vi "Read controlTerminalRef.vi"(8 "error in (no error)":errorcluster, 11 "Terminal In":refnum<class "ControlTerminal.lvclass">) -> (0 "error out":errorcluster, 2 "terminalRef":refnum<vi>, 3 "Terminal Out":refnum<class "ControlTerminal.lvclass">)   [LabVIEW 2023, in "TLC_Scripto.lvlib" / "ControlTerminal.lvclass"]
uses:
  ControlTerminal.lvclass
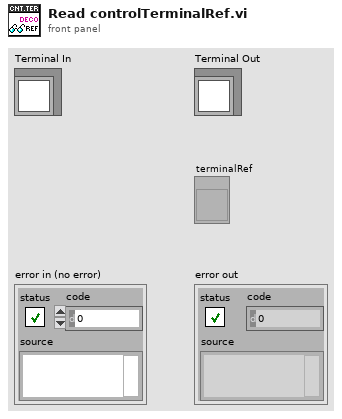
[diagram p1: front panel]
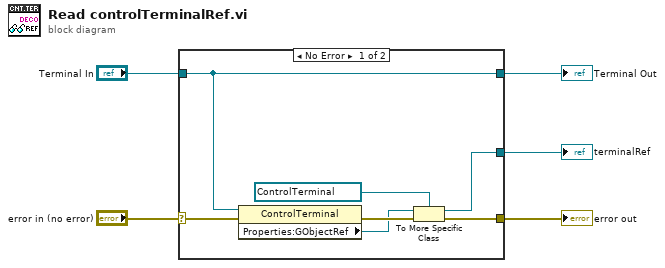
[diagram p0: block diagram]
diagram:
  n1 = case shown="No Error" "error in (no error)" {
    selector: "error in (no error)" -> [w9 w14]
    tunnel: [w8 w14] -> w4
    tunnel: [w10 w13] -> w2
    tunnel: "Terminal In" -> [w10 w13]
    tunnel: [w7 _] -> w1
    frame No Error {
      n2 = property class="ControlTerminal"(reference=w10, error in=w9) -> (error out=w12:errorcluster, "Properties:GObjectRef"=w11:refnum<vi>)  [unwired: 1 out]
      n3 = To More Specific Class(target class=refnum<vi> refnum ("terminalRef"), reference=w11, error in=w12) -> (specific class reference=w7:refnum<vi>, error out=w8:errorcluster)
    }
    frame Error {
    }
  }
  "error out" <- w4
  "Terminal Out" <- w2
  "terminalRef" <- w1
